vi "mclustBIC.vi"() -> ()   [LabVIEW 2014]
panel:
  in  "modelName":string
  in  "G":dbl[](array[numeric])
  in  "data":dbl[][](array[numeric])=[[0.0, 0.0], [0.0, 0.0], [0.0, 0.0], [0.0, 0.0], [0.0, 0.0], [0.0, 0.0], [0.0, -1.0]]
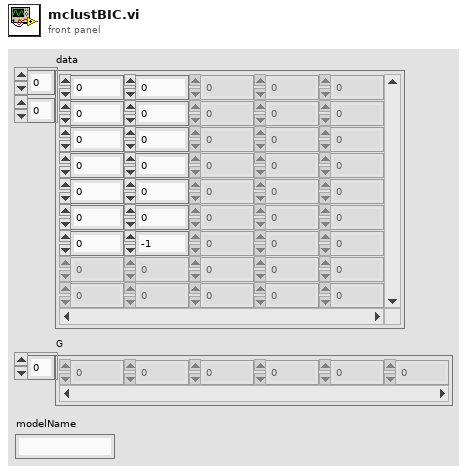
[diagram p1: front panel]
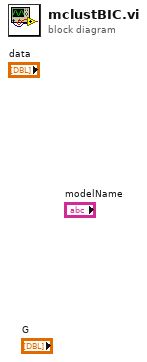
[diagram p0: block diagram]
diagram:
